vi "Read functions.vi"(8 "error in":errorcluster, 11 "Logic Sequencer configuration in":refnum<class "Logic Sequencer configuration.lvclass">) -> (0 "error out":errorcluster, 2 "functions":T1[](array[typedef]), 3 "Logic Sequencer configuration out":refnum<class "Logic Sequencer configuration.lvclass">)   [LabVIEW 2013, in "Logic Sequencer configuration.lvclass"]
uses:
  Logic Sequencer configuration.lvclass
  processing channels.ctl
  <vilib>/NI/Tag Bus Module Framework/channel/TBM channel.lvclass
  Logic Sequencer configuration.lvclass/Logic Sequencer configuration.ctl
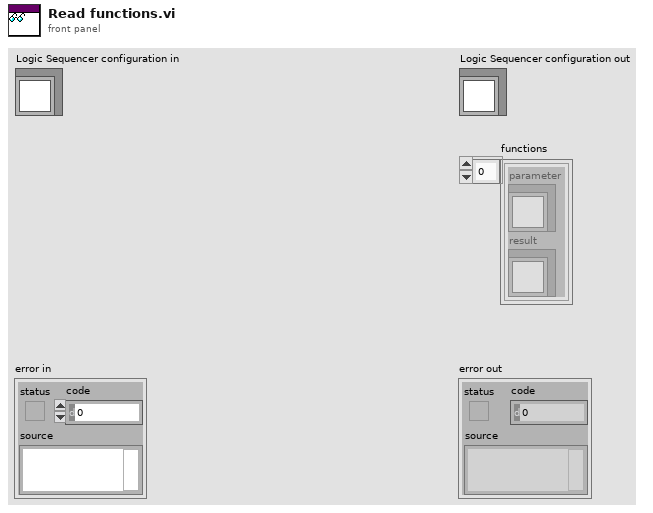
[diagram p1: front panel]
types:
  T1 = typedef "Logic Sequencer configuration.lvclass/processing channels.ctl" = cluster{"parameter":refnum<class "TBM channel.lvclass">, "result":refnum<class "TBM channel.lvclass">}
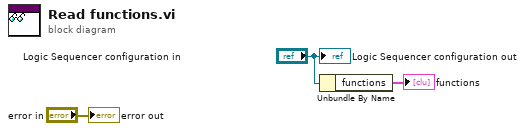
[diagram p0: block diagram]
diagram:
  n1 = Unbundle By Name("Logic Sequencer configuration in") -> ("functions"=→"functions":T1[])
  "error out" <- "error in"
  "Logic Sequencer configuration out" <- "Logic Sequencer configuration in"
